vi "calculatePsrrRawWfms.vi"(6 "Time signal(s) in":waveform(dbl)[](array[waveform]), 8 "error in (no error)":errorcluster, 9 "Calculation method":enum16{"RMS", "Peak-to-peak"}(ring), 10 "Search frequency":dbl, 11 "Instrument handle":refnum<k15>) -> (0 "error out":errorcluster, 1 "Detected wfm parameters":T2, 2 "PSRR":dbl, 3 "Instrument handle out":refnum<k15>, 4 "Detected signal(s)":T1(array[cluster]) {"exported spectrum (dB)"."dB Spectrum (Hann)" format="%.2p"; "exported spectrum (dB)"."df" format="%.2p"; "exported spectrum (dB)"."f0" format="%.2p"})   [LabVIEW 2020]
uses:
  <vilib>/measure/matone.llb/Extract Single Tone Information N Chan.vi
  <vilib>/measure/madcrms.llb/Basic Averaged DC-RMS for N Chan.vi
  <vilib>/measure/mascope.llb/Amplitude and Levels N chan.vi
  <vilib>/measure/NI_MAPro.lvlib
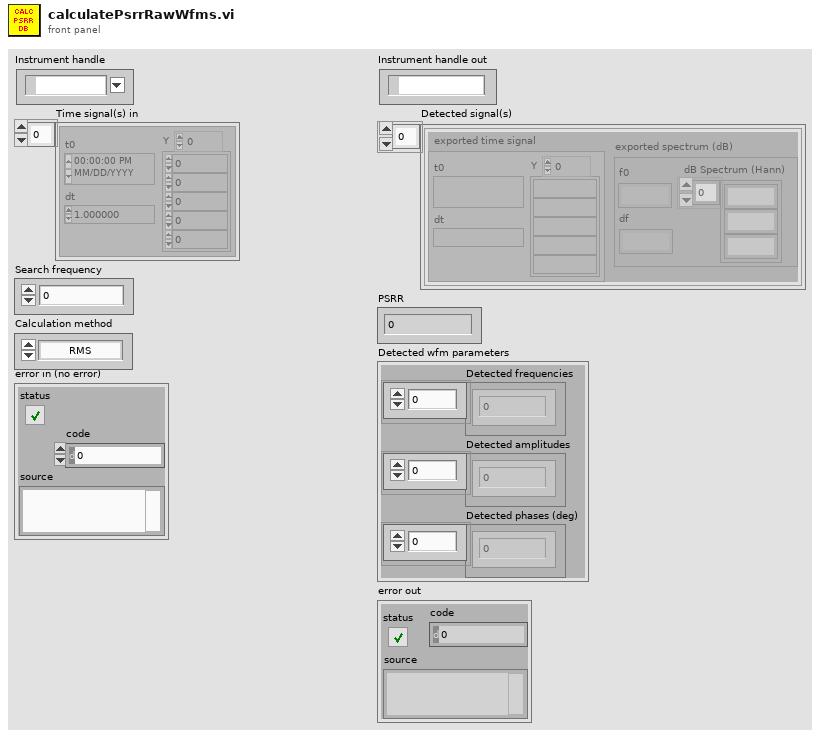
[diagram p1: front panel]
types:
  T1 = cluster{"exported time signal":waveform(dbl), "exported spectrum (dB)":cluster{"f0":dbl, "df":dbl, "dB Spectrum (Hann)":dbl[]}}[]
  T2 = cluster{"Detected frequencies":dbl[], "Detected amplitudes":dbl[], "Detected phases (deg)":dbl[]}
  T3 = enum32{"none", "input signal", "detected signal", "residual signal"}
  T4 = cluster{"Search frequency":dbl, "search (+/- % of Fsampl.)":dbl}
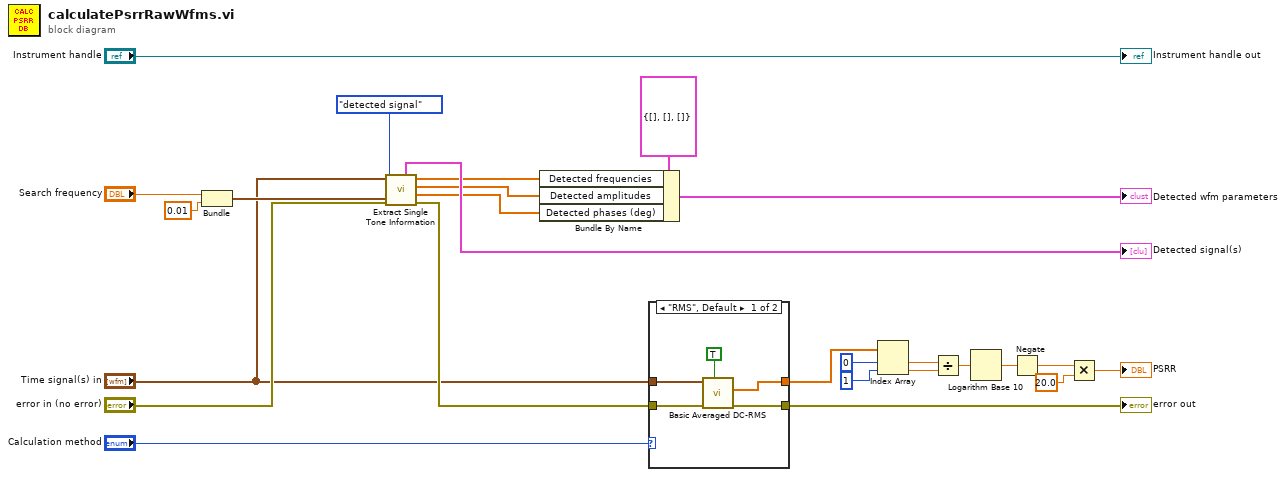
[diagram p0: block diagram]
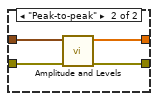
[diagram p2: hidden frame]
diagram:
  n1 = Bundle("Search frequency"="Search frequency", "search (+/- % of Fsampl.)"=0.01) -> (w23:T4)  [unwired: 1 in]
  n2 = call-poly <vilib>:"Extract Single Tone Information.vi"("advanced search"=w23, "error in (no error)"="error in (no error)", "export mode"=T3."detected signal", "time signals in"="Time signal(s) in") -> ("error out"=w15:errorcluster, "detected phases (deg)"=w19:dbl[], "detected amplitudes"=w20:dbl[], "detected frequencies"=w21:dbl[], "exported signals"=→"Detected signal(s)":T1)  [unwired: 2 in, 1 out]
  n3 = Bundle By Name(cluster=T2 {"Detected frequencies"=[], "Detected amplitudes"=[], "Detected phases (deg)"=[]} ("input cluster"), "Detected frequencies"=w21, "Detected amplitudes"=w20, "Detected phases (deg)"=w19) -> (→"Detected wfm parameters":T2)
  n4 = case shown="\"RMS\", Default" "Calculation method" {
    tunnel: w15 -> [w31 w34]
    tunnel: [w30 w32] -> w14
    tunnel: "Time signal(s) in" -> [w29 w35]
    tunnel: [w27 w33] -> w13
    frame "RMS", Default {
      n5 = call-poly <vilib>:"Basic Averaged DC-RMS.vi"("reset"=TRUE, "error in (no error)"=w31, "signals in"=w29) -> ("error out"=w30:errorcluster, "RMS values"=w27:dbl[])  [unwired: 5 in, 2 out]
    }
    frame "Peak-to-peak" {
      n6 = call-poly <vilib>:"Amplitude and Levels.vi"("error in (no error)"=w34, "signal(s) in"=w35) -> ("error out"=w32:errorcluster, "amplitude"=w33:dbl[])  [unwired: 6 in, 2 out]
    }
  }
  "error out" <- w14
  n7 = Index Array(array=w13, index #1=0 ("index"), index #2=1 ("index")) -> (element #1=w9:dbl, element #2=w10:dbl)
  n8 = Divide(x=w9, y=w10) -> (x/y=w8:dbl)
  n9 = Logarithm Base 10(1:w8) -> (0:w7:dbl)
  n10 = Negate(x=w7) -> (-x=w3:dbl)
  n11 = Multiply(x=w3, y=20.0) -> (x*y=→"PSRR":dbl)
  "Instrument handle out" <- "Instrument handle"
